vi "Test_Photoresistor.vi"() -> ()   [LabVIEW 2017]
uses:
  <vilib>/express/express analysis/Spectral/Block/exnSpectralBlock spectral measurements RMS poly.vi
  <vilib>/express/express analysis/Spectral/Block/exnSpectralBlock spectral measurements RMS DDT.vi
  <vilib>/measure/maspectr.llb/FFT Spectrum (Mag-Phase) for 1 Chan.vi
  <vilib>/express/express analysis/Spectral/XNode/ExpressSpectralMeasurementsBlockNode.xnode
  <vilib>/measure/NI_MAPro.lvlib
panel:
  out "Spectrum":dynamicdata(graph)
  out "magnitude":cluster{"f0":dbl, "df":dbl, "magnitude":dbl[]}(graph)
  out "Waveform Chart":i32[](graph)
  in  "stop":bool
  in  "Samples qty":i32
  in  "Period (ms)":u32=10
  in  "COM Port":refnum<visa-resource-name>="COM1"
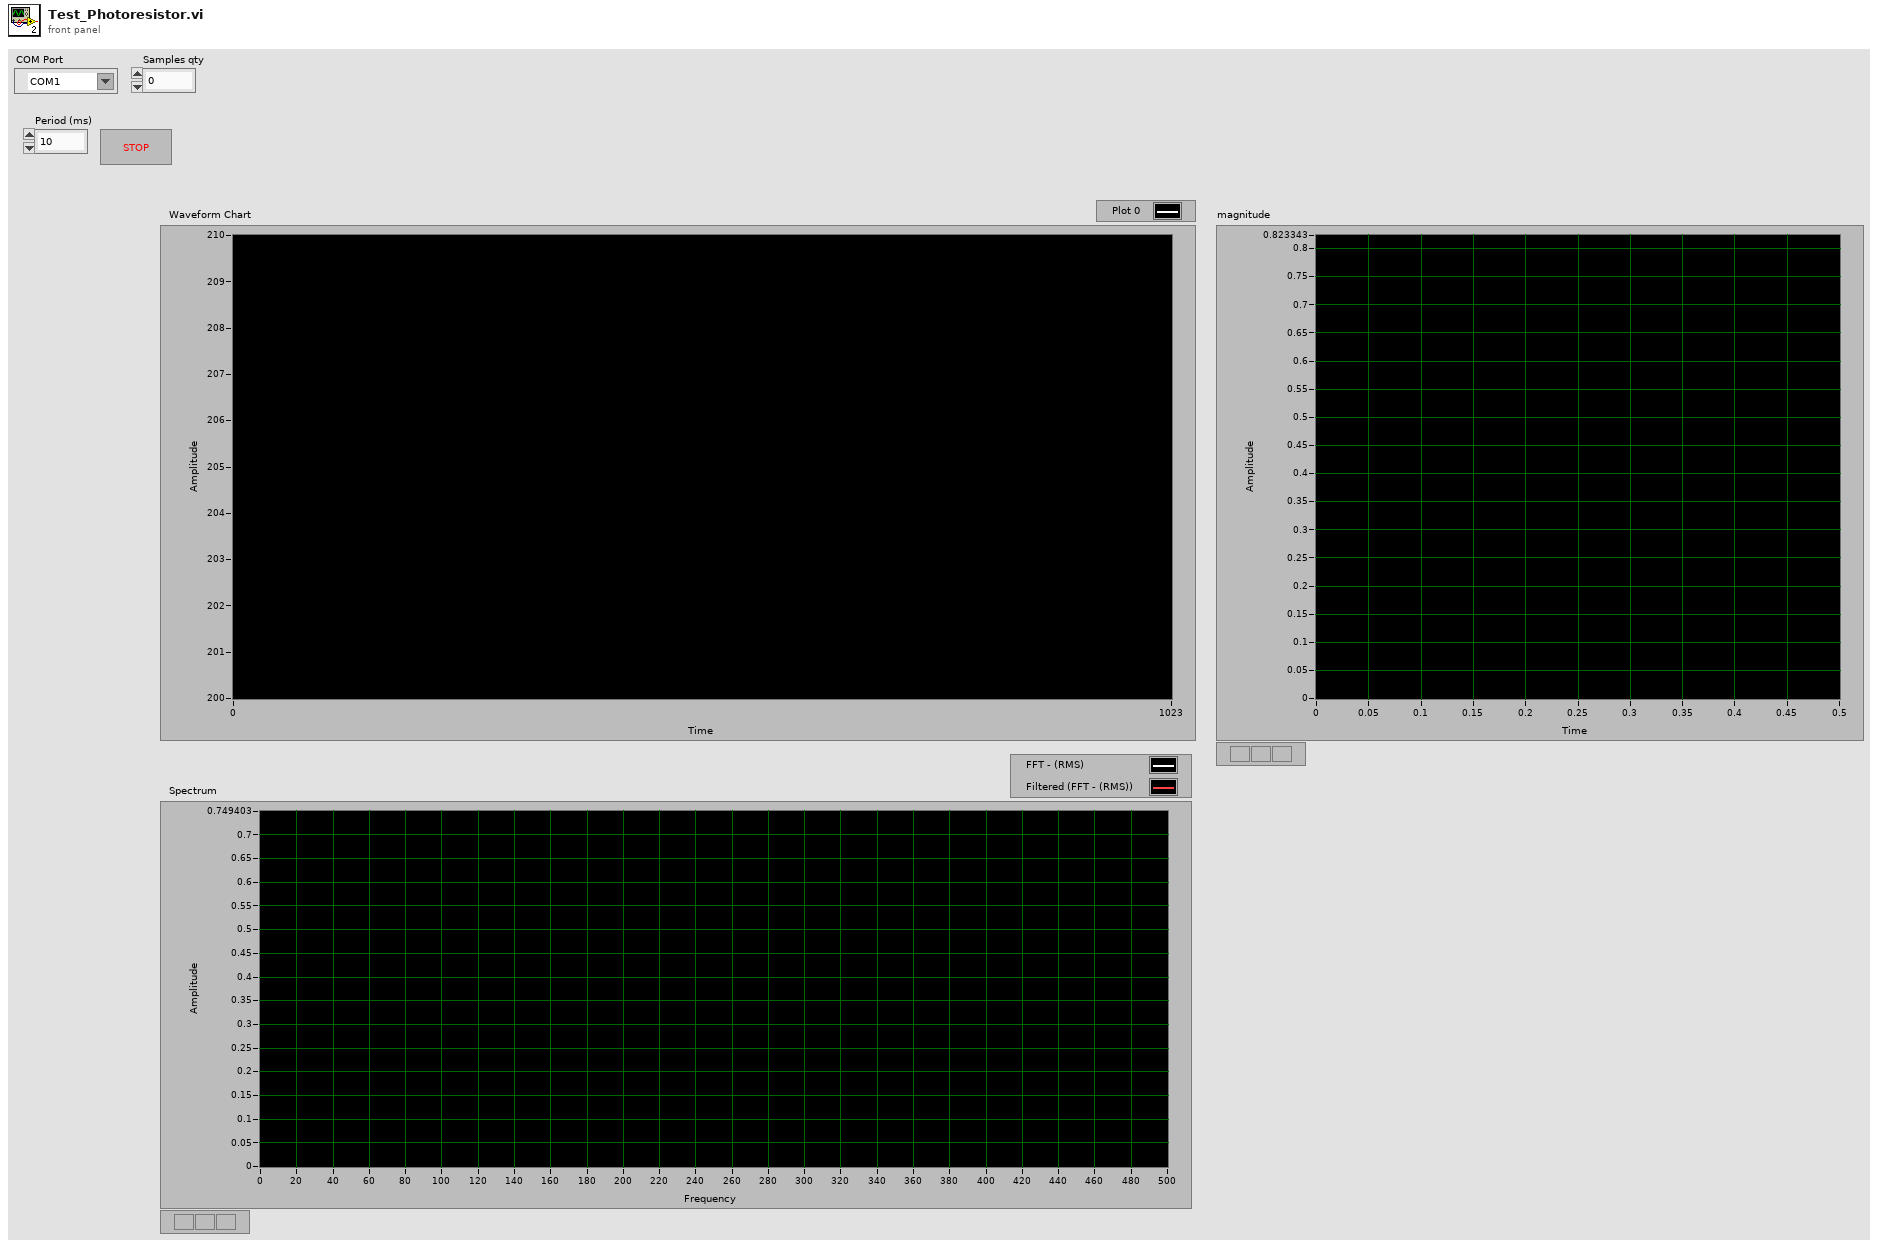
[diagram p1: front panel]
types:
  T1 = cluster{"averaging mode":u16, "weighting mode":u16, "number of averages":u32}
  T2 = cluster{"dB On (F)":bool, "unwrap phase (F)":bool, "convert to degree (F)":bool}
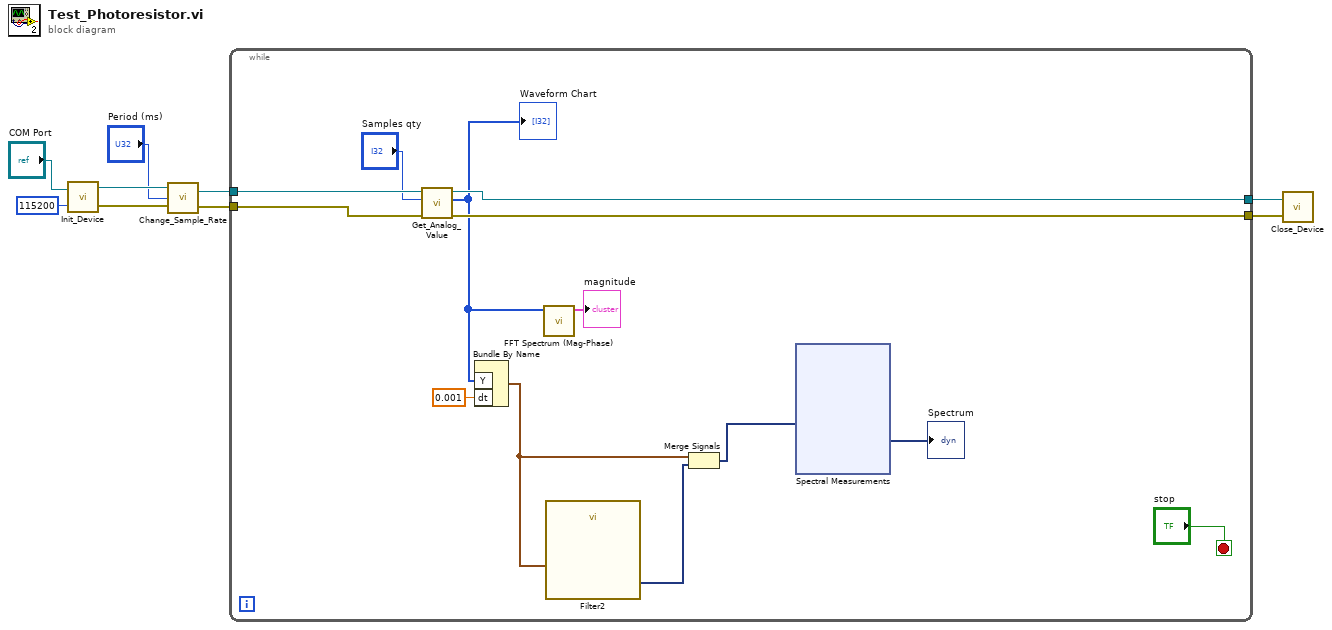
[diagram p0: block diagram]
diagram:
  n1 = call "Init_Device.vi"("Baud Rate"=u32 115200, "COM Port"="COM Port") -> ("error out"=w6:errorcluster, "Device Session"=w7:refnum<visa-resource-name>)
  n2 = call "Change_Sample_Rate.vi"("error in"=w6, "Period (ms)"="Period (ms)", "Device Session In"=w7) -> ("error out"=w5:errorcluster, "Device Session Out"=w4:refnum<visa-resource-name>)
  n3 = while {
    tunnel: w5 -> [w22]
    tunnel: w4 -> [w21]
    tunnel: [w18] -> w2
    tunnel: [w17] -> w1
    stop <- "stop" stop-if-true
    n4 = call "Get_Analog_Value.vi"("error in"=w22, "Samples qty"="Samples qty", "Device Session In"=w21) -> ("error out"=w18:errorcluster, "Output values"=w13:i32[], "Device Session Out"=w17:refnum<visa-resource-name>)  [unwired: 5 in]
    "Waveform Chart" <- w13
    n5 = Bundle By Name("Y"=w13, "dt"=0.001) -> (w12:waveform(i32))  [unwired: 1 in]
    n6 = call-poly <vilib>:"FFT Spectrum (Mag-Phase).vi"("time signal"=w13) -> ("magnitude"=→"magnitude":cluster{"f0":dbl, "df":dbl, "magnitude":dbl[]})  [unwired: 6 in, 4 out]
    n7 = call "Filter2"("Signal"=w12) -> ("Filtered Signal"=w10:dynamicdata)  [unwired: 9 in, 1 out]
    n8 = Merge Signals(w12, w10) -> (w11:dynamicdata)
    n9 = xnode "Spectral Measurements"("Signals"=w11) -> ("FFT - (RMS)"=→"Spectrum":dynamicdata)  [unwired: 1 in, 2 out]
  }
  n10 = call "Close_Device.vi"("error in"=w2, "Device Session"=w1) -> ()  [unwired: 1 in, 1 out]
